vi "Create User Events.vi"(11 "Cooler UI with Events in":refnum<class "Cooler UI with Events.lvclass">=refnum) -> (2 "Events":T1, 3 "Cooler UI with Events out":refnum<class "Cooler UI with Events.lvclass">)   [LabVIEW 2012]
uses:
  Status.ctl
  Cooler UI with Events.lvclass
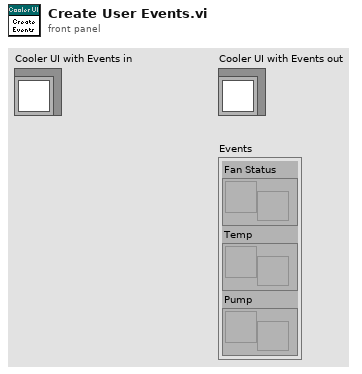
[diagram p1: front panel]
types:
  T1 = cluster{"Fan Status":refnum<user-event>, "Temp":refnum<user-event>, "Pump":refnum<user-event>}
  T2 = typedef "Cooler UI.lvlib/Cooler UI with Events.lvclass/Status.ctl" = cluster{"Fan A":cluster{"State":bool, "Fault":bool}, "Fan B":cluster{"State":bool, "Fault":bool}}
  T3 = cluster{"Fan Status":refnum<user-event>, "Temperature":refnum<user-event>, "Pump":refnum<user-event>}
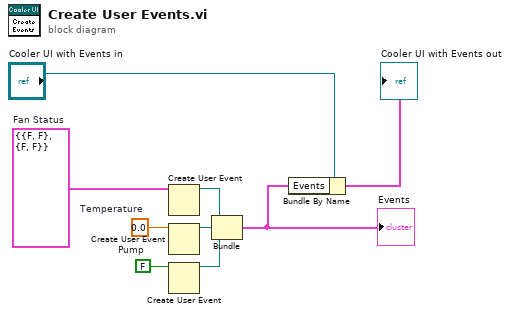
[diagram p0: block diagram]
diagram:
  w1 = T2 {"Fan A"={"State"=FALSE, "Fault"=FALSE}, "Fan B"={"State"=FALSE, "Fault"=FALSE}}  # Fan Status
  w6 = FALSE  # Pump
  w5 = 0.0  # Temperature
  n1 = Create User Event(user event datatype=w1) -> (user event=w7:refnum<user-event>)  [unwired: 1 in, 1 out]
  n2 = Create User Event(user event datatype=w5) -> (user event=w8:refnum<user-event>)  [unwired: 1 in, 1 out]
  n3 = Create User Event(user event datatype=w6) -> (user event=w9:refnum<user-event>)  [unwired: 1 in, 1 out]
  n4 = Bundle("Fan Status"=w7, "Temperature"=w8, "Pump"=w9) -> (w2:T3)  [unwired: 1 in]
  "Events" <- w2
  n5 = Bundle By Name(cluster="Cooler UI with Events in", "Events"=w2) -> (→"Cooler UI with Events out":cluster{})
